vi "TC560-Buzzer.vi"(8 "error in":errorcluster, 9 "Sound Volume":T1(ring), 10 "Command":T2(ring), 11 "VISA Resource Name In":refnum<visa-resource-name>) -> (0 "error out":errorcluster, 3 "VISA Resource Name Out":refnum<visa-resource-name>)   [LabVIEW 2018]
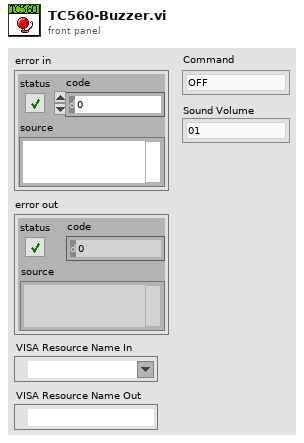
[diagram p1: front panel]
types:
  T1 = enum16{"01", "02", "03", "04", "05", "06", "07", "08", "09", "10"}
  T2 = enum16{"OFF", "GO", "HI", "LO", "HILO", "PASS", "FAIL", "GOOD", "NG"}
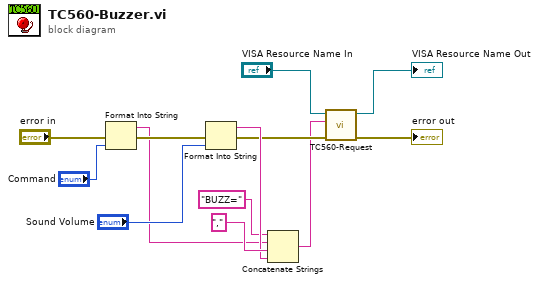
[diagram p0: block diagram]
diagram:
  n1 = Format Into String(error in="error in", "Command") -> (resulting string=w1:string, error out=w4:errorcluster)  [unwired: 2 in]
  n2 = Format Into String(error in=w4, "Sound Volume") -> (resulting string=w12:string, error out=w9:errorcluster)  [unwired: 2 in]
  n3 = Concatenate Strings("BUZZ=" ("string"), w1, "," ("string"), w12) -> (w8:string)
  n4 = call "TC560-Request.vi"("error in"=w9, "Command"=w8, "VISA Resource Name In"="VISA Resource Name In") -> ("error out"=→"error out":errorcluster, "VISA Resource Name Out"=→"VISA Resource Name Out":refnum<visa-resource-name>)  [unwired: 6 in, 1 out]
